vi "Priority.vi"(8 "error in (no error)":errorcluster, 11 "Test Index in":refnum<class "Test Index.lvclass">) -> (0 "error out":errorcluster, 2 "Priority":u16, 3 "Test Index out":refnum<class "Test Index.lvclass">)   [LabVIEW 2020]
uses:
  Test Index.lvclass
  Test Index.lvclass/Test Index.ctl
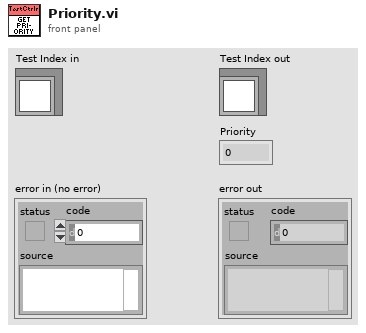
[diagram p1: front panel]
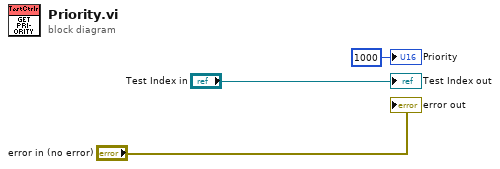
[diagram p0: block diagram]
diagram:
  "error out" <- "error in (no error)"
  "Test Index out" <- "Test Index in"
  "Priority" <- u16 1000 ("Priority")
